vi "SERF Field Monitor.vi"() -> ()   [LabVIEW 2017]
uses:
  <instrlib>/tio-labview/Labview Signal Processing/Log Binning.vi
  <vilib>/Utility/error.llb/Clear Errors.vi
  <instrlib>/tio-labview/Labview Signal Processing/Log Range.vi
  <instrlib>/tio-labview/TIO Library/Data Stream/TIO Data Stream Parse Description.vi
  <vilib>/Utility/file.llb/Write Delimited Spreadsheet (DBL).vi
  <vilib>/Analysis/6fits.llb/General Polynomial Fit.vi
  <vilib>/measure/maspectr.llb/FFT Power Spectrum and PSD.vi
  <vilib>/measure/maspectr.llb/FFT Power Spectrum and PSD for 1 Chan.vi
panel:
  in  "Log":bool
  in  "Log to file":path
  in  "Zero":bool
  out "Status":bool[](array[boolean])
  in  "Enable Z":bool
  in  "Enable Y":bool
  in  "Calibrate":bool
  out "Kill":bool=TRUE
  in  "Quit":bool
  in  "Reset":bool
  in  "Duration":dbl[unit]=100.0
  in  "URL":refnum<visa-resource-name>="tcp://localhost"
  out "Y":cluster{dbl, dbl, dbl[][]}(graph)={3358.7436, 0.0012, []}
  in  "Bin":bool=TRUE
  out "XY Graph":T1(graph)
  # "SERF \nVector Magnetometer"
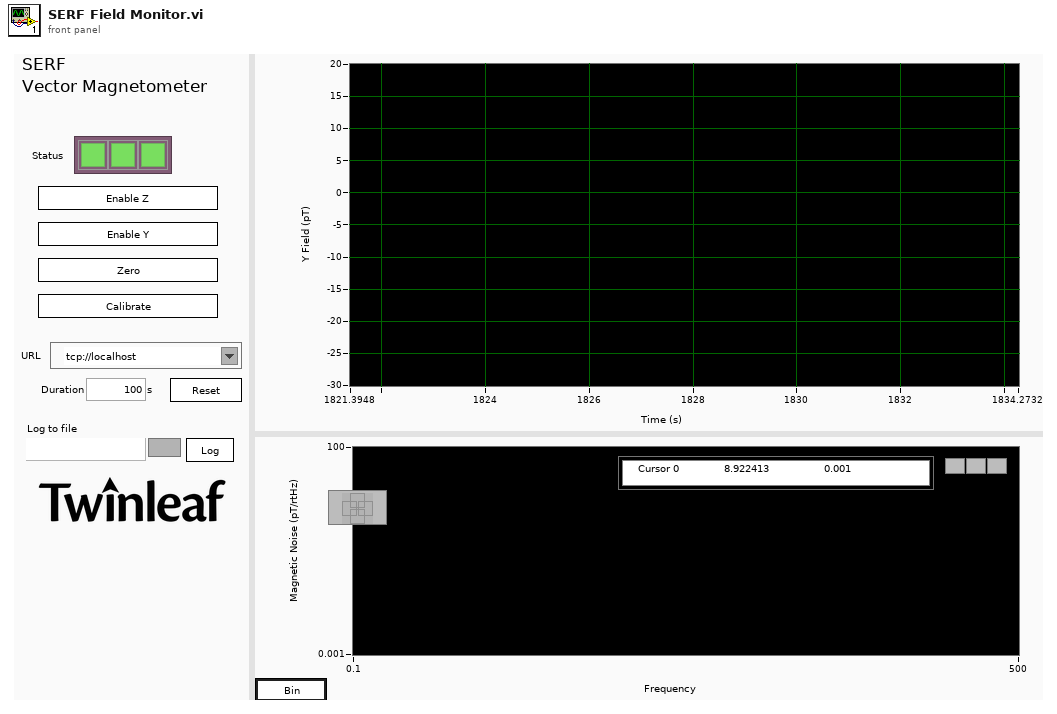
[diagram p1: front panel]
types:
  T1 = cluster{"Frequencies Binned":dbl[], "Spectrum Binned":dbl[]}[]
  T2 = cluster{"Type":enum16{"TCP", "Serial"}, "Serial":refnum<visa-resource-name>, "TCP":refnum<k5>, "Timeout":u32}
  T3 = cluster{"Stream Description":cluster{"Stream ID":u16, "Data Type":u8, "Channels":u8, "Restart ID":u16, "Start timestamp (s)":dbl, "Sample counter":u64, "Period (s)":dbl, "Flags":u8, "Timestamp type":u8, "Name":string, "Last sample number":u64, "Last Restart ID":u16, "Version":u16, "Sample Size":u16}, "Sample #":u32, "Raw Data":string}
  T4 = cluster{"Frequencies Binned":dbl[], "Spectrum Binned":dbl[]}
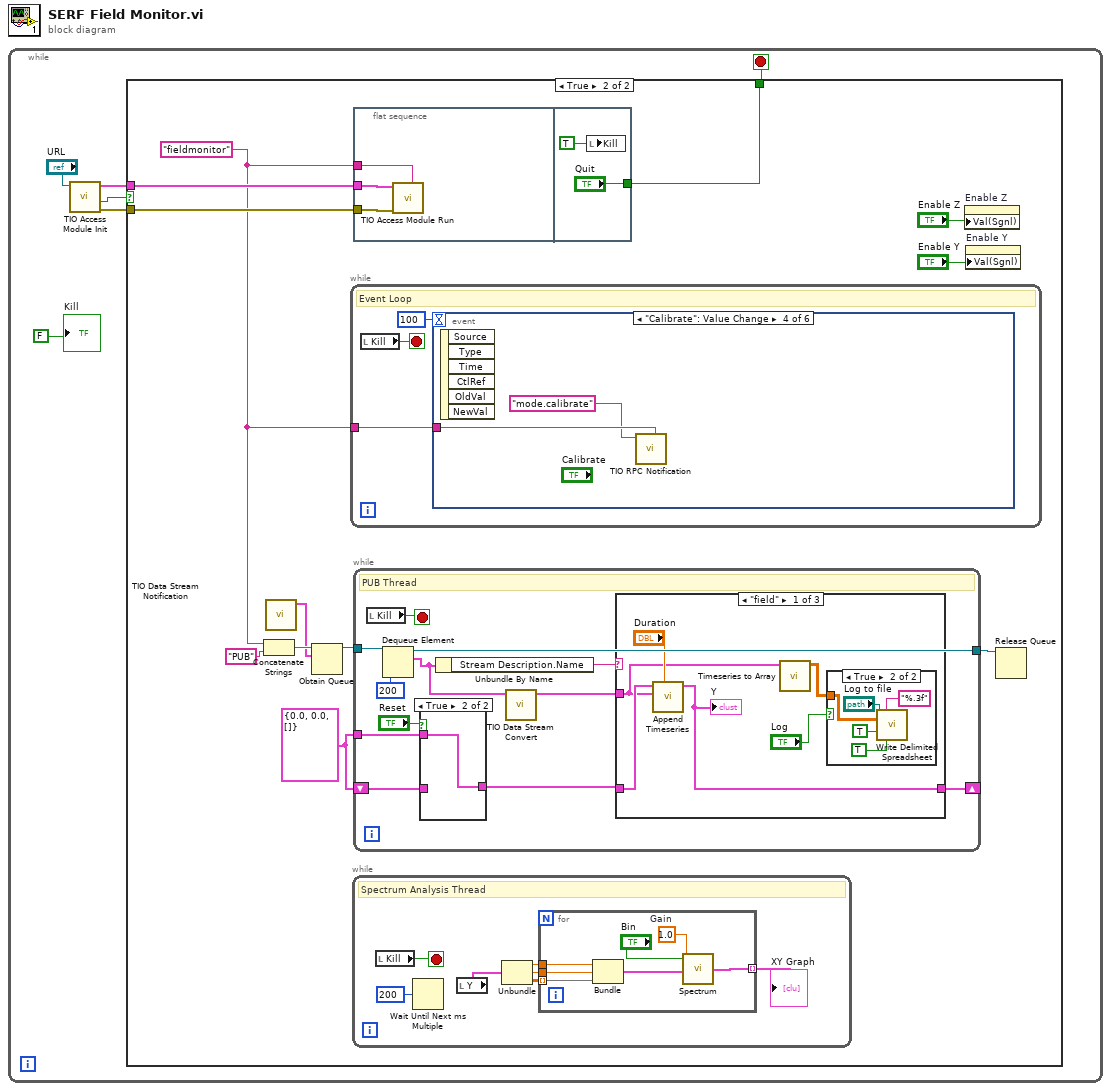
[diagram p0: block diagram]
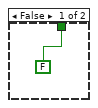
[diagram p2: hidden frame]
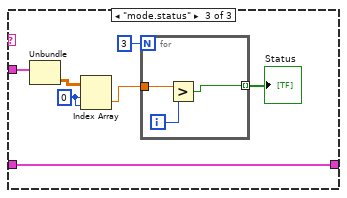
[diagram p6: hidden frame]
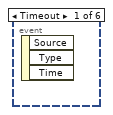
[diagram p7: hidden frame]
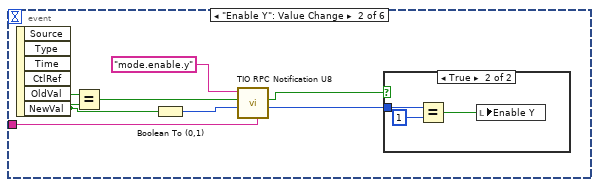
[diagram p8: hidden frame]
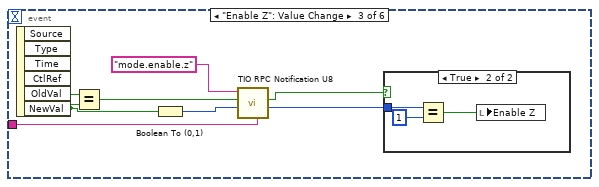
[diagram p10: hidden frame]
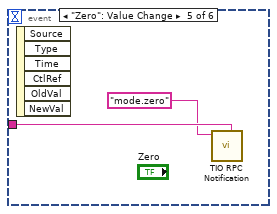
[diagram p12: hidden frame]
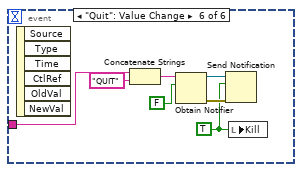
[diagram p13: hidden frame]
diagram:
  n1 = while {
    stop <- w6 stop-if-true
    n2 = call <instrlib>:"TIO Access Module Init.vi"("URL"="URL") -> ("error out"=w2:errorcluster, "Connected"=w1:bool, "TS Connection"=w3:T2)  [unwired: 8 in]
    n3 = case shown="True" w1 {
      tunnel: [FALSE ("Quit") w13] -> w6
      tunnel: w3 -> [_ w12]
      tunnel: w2 -> [_ w11]
      frame False {
      }
      frame True {
        w10 = "fieldmonitor" ("Coil")
        w15 = cluster{dbl, dbl, dbl[][]} {0.0, 0.0, []} ("Waveform Timeseries")
        n4 = Concatenate Strings(w10, "PUB" ("name (unnamed)")) -> (w19:string)
        n5 = call <instrlib>:"TIO Data Stream Notification.vi"() -> ("Data Stream Notification"=w14:T3)  [unwired: 11 in]
        n6 = Obtain Queue(name (unnamed)=w19, element data type=w14) -> (queue out=w17:refnum<queue>)  [unwired: 3 in, 2 out]
        n7 = while {
          tunnel: w10 -> [w75]
          stop <- w77 stop-if-true
          # "Event Loop"
          n8 = local read "Kill"() -> (w77:bool)
          n9 = event shown="[3] \"Calibrate\": Value Change" {
            selector: _ -> [_ _ _ _ _ _]
            dyn-events: _ -> [_ _ _ _ _ _]
            timeout: 100 -> [_ _ _ _ _ _]
            tunnel: w75 -> [_ w82 w93 w101 w103 w104]
            event Timeout {
              n10 = event-data() -> ()  [unwired: 1 in, 3 out]
            }
            event "Enable Y": Value Change {
              n11 = event-data() -> ("OldVal"=w85:bool, "NewVal"=w79:bool)  [unwired: 1 in, 4 out]
              n12 = Equal?(x=w85, y=w79) -> (x = y?=w84:bool)
              n13 = Boolean To (0,1)(Boolean=w79) -> (0, 1=w83:i16)
              n14 = call <instrlib>:"TIO RPC Notification U8.vi"("Notification Prefix"=w82, "U8"=w83, "Read"=w84, "String"="mode.enable.y" ("Topic")) -> ("U8"=w80:u8, "Response"=w81:bool)  [unwired: 4 in, 1 out]
              n15 = case shown="True" w81 {
                tunnel: w80 -> [_ w88]
                frame False {
                }
                frame True {
                  n16 = Equal?(x=w88, y=u8 1) -> (x = y?=w86:bool)
                  n17 = local write "Enable Y"(w86) -> ()
                }
              }
            }
            event "Enable Z": Value Change {
              n18 = event-data() -> ("OldVal"=w96:bool, "NewVal"=w90:bool)  [unwired: 1 in, 4 out]
              n19 = Equal?(x=w96, y=w90) -> (x = y?=w95:bool)
              n20 = Boolean To (0,1)(Boolean=w90) -> (0, 1=w94:i16)
              n21 = call <instrlib>:"TIO RPC Notification U8.vi"("Notification Prefix"=w93, "U8"=w94, "Read"=w95, "String"="mode.enable.z" ("Topic")) -> ("U8"=w91:u8, "Response"=w92:bool)  [unwired: 4 in, 1 out]
              n22 = case shown="True" w92 {
                tunnel: w91 -> [_ w99]
                frame False {
                }
                frame True {
                  n23 = Equal?(x=w99, y=u8 1) -> (x = y?=w97:bool)
                  n24 = local write "Enable Z"(w97) -> ()
                }
              }
            }
            event "Calibrate": Value Change {
              n25 = event-data() -> ()  [unwired: 1 in, 6 out]
              n26 = call <instrlib>:"TIO RPC Notification.vi"("Notification Prefix"=w101, "Topic"="mode.calibrate") -> ()  [unwired: 6 in, 3 out]
            }
            event "Zero": Value Change {
              n27 = event-data() -> ()  [unwired: 1 in, 6 out]
              n28 = call <instrlib>:"TIO RPC Notification.vi"("Notification Prefix"=w103, "Topic"="mode.zero") -> ()  [unwired: 6 in, 3 out]
            }
            event "Quit": Value Change {
              w105 = TRUE ("Kill")
              n29 = event-data() -> ()  [unwired: 1 in, 6 out]
              n30 = Concatenate Strings(w104, "QUIT" ("name (unnamed)")) -> (w110:string)
              n31 = Obtain Notifier(name (unnamed)=w110, notification data type=FALSE ("Connected")) -> (notifier out=w107:refnum<notifier>, error out=w108:errorcluster)  [unwired: 2 in, 1 out]
              n32 = Send Notification(notification=w105, notifier=w107, error in (no error)=w108) -> ()  [unwired: 2 out]
              n33 = local write "Kill"(w105) -> ()
            }
          }
        }
        n34 = while {
          stop <- w25 stop-if-true
          # "Spectrum Analysis Thread"
          n35 = local read "Kill"() -> (w25:bool)
          n36 = Wait Until Next ms Multiple(millisecond multiple=u32 200) -> ()  [unwired: 1 out]
          n37 = local read "Y"() -> (w23:cluster{dbl, dbl, dbl[][]})
          n38 = Unbundle(w23) -> (w21:dbl, w20:dbl, w22:dbl[][])
          n39 = for {
            tunnel: [w33] -> w24 mode=indexing
            tunnel: w22 -> [w27] mode=indexing
            tunnel: w21 -> [w29]
            tunnel: w20 -> [w28]
            w31 = 1.0  # Gain
            n40 = Bundle(w29, w28, w27) -> (w30:cluster{dbl, dbl, dbl[]})  [unwired: 1 in]
            n41 = call <instrlib>:"Spectrum.vi"("Gain"=w31, "Waveform 1"=w30, "Binning"="Bin") -> ("Cluster"=w33:T4)  [unwired: 2 in]
          }
          "XY Graph" <- w24
        }
        n42 = flat-sequence {
          tunnel: w10 -> [w72]
          tunnel: w12 -> [w71]
          tunnel: w11 -> [w70]
          tunnel: ["Quit"] -> w13
          frame #0 {
            n43 = call <instrlib>:"TIO Access Module Run.vi"("Notification Prefix"=w72, "error in (no error)"=w70, "TS Connection"=w71) -> ()  [unwired: 9 in]
          }
          frame #1 {
            n44 = local write "Kill"(TRUE ("Kill")) -> ()
          }
        }
        n45 = while {
          tunnel: w17 -> [w44]
          shift-right: [w43] -> _
          shift-left: w15 -> [w41]
          tunnel: w15 -> [w40]
          tunnel: [w37] -> w16
          stop <- w45 stop-if-true
          # "PUB Thread"
          n46 = local read "Kill"() -> (w45:bool)
          n47 = Dequeue Element(queue=w44, timeout in ms (-1)=200) -> (queue out=w37:refnum<queue>, element=w36:T3)  [unwired: 1 in, 2 out]
          n48 = case shown="True" "Reset" {
            tunnel: w41 -> [w46 _]
            tunnel: [w46 w47] -> w39
            tunnel: w40 -> [_ w47]
            frame False {
            }
            frame True {
            }
          }
          n49 = Unbundle By Name(w36) -> ("Stream Description.Name"=w34:string)
          n50 = call <instrlib>:"TIO Data Stream Convert.vi"("Data Stream Notification"=w36) -> ("Waveform"=w35:cluster{dbl, dbl, dbl[][]})  [unwired: 10 in]
          n51 = case shown="\"field\"" w34 {
            tunnel: [w52 w59 w66] -> w43
            tunnel: w39 -> [w53 w59 w66]
            tunnel: w35 -> [w49 _ w65]
            frame "field" {
              n52 = call <instrlib>:"Append Timeseries.vi"("Duration"="Duration", "Waveform New"=w49, "Waveform History"=w53) -> ("Waveform Timeseries"=w52:cluster{dbl, dbl, dbl[][]})  [unwired: 8 in]
              "Y" <- w52
              n53 = call <instrlib>:"Timeseries to Array.vi"("Waveform New"=w49) -> (3:w48:dbl[][])  [unwired: 10 in]
              n54 = case shown="True" "Log" {
                tunnel: w48 -> [_ w58]
                frame False {
                }
                frame True {
                  n55 = call-poly <vilib>:"Write Delimited Spreadsheet.vi"("file path (dialog if empty)"="Log to file", "format (%.3f)"="%.3f", "2D data"=w58, "append to file? (new file:F)"=TRUE ("append to file? (F)"), "transpose? (no:F)"=TRUE ("transpose? (F)")) -> ()  [unwired: 9 in, 2 out]
                }
              }
            }
            frame Default {
            }
            frame "mode.status" {
              w63 = 0 ("index (row)")
              n56 = Unbundle(w65) -> (w64:dbl[][])  [unwired: 2 out]
              n57 = Index Array(array=w64, index (row)=w63, index (col)=w63) -> (element=w62:dbl)
              n58 = for {
                N: 3 -> [_]
                tunnel: w62 -> [w69]
                tunnel: [w67] -> w61 mode=indexing
                i -> [w68]
                n59 = Greater?(x=w69, y=w68) -> (0:w67:bool)
              }
              "Status" <- w61
            }
          }
        }
        n60 = property on="Enable Z" class="Bool (strict)"("Val(Sgnl)"="Enable Z") -> ()  [unwired: 2 in, 2 out]
        n61 = property on="Enable Y" class="Bool (strict)"("Val(Sgnl)"="Enable Y") -> ()  [unwired: 2 in, 2 out]
        n62 = Release Queue(queue=w16) -> ()  [unwired: 2 in, 3 out]
      }
    }
    "Kill" <- FALSE ("Kill")
  }
